vi "GapDetectionNew_nextFour_BM_markus_4.vi"(8 "Sigma in Prozent":dbl=3.0, 9 "Gap":dbl=85.0, 11 "Locations":dbl[](array[numeric])=[1075.5115609583977, 1096.8761989990003, 1148.4828033713086, 1170.9683288122183, 1215.5424277113636]) -> (0 "distanceMatrix":dbl[][](array[numeric])=[[21.364638040602586]], 1 "Array":dbl[](array[numeric]), 2 "FirstGap":dbl=21.364638040602586, 3 "GapPresent":bool)   [LabVIEW 2014]
panel:
  in  "Number of following reflections that should be regarded":i32=1
  in  "probaility higher than":dbl=0.7
  out "exp(x)":dbl[][](array[numeric])
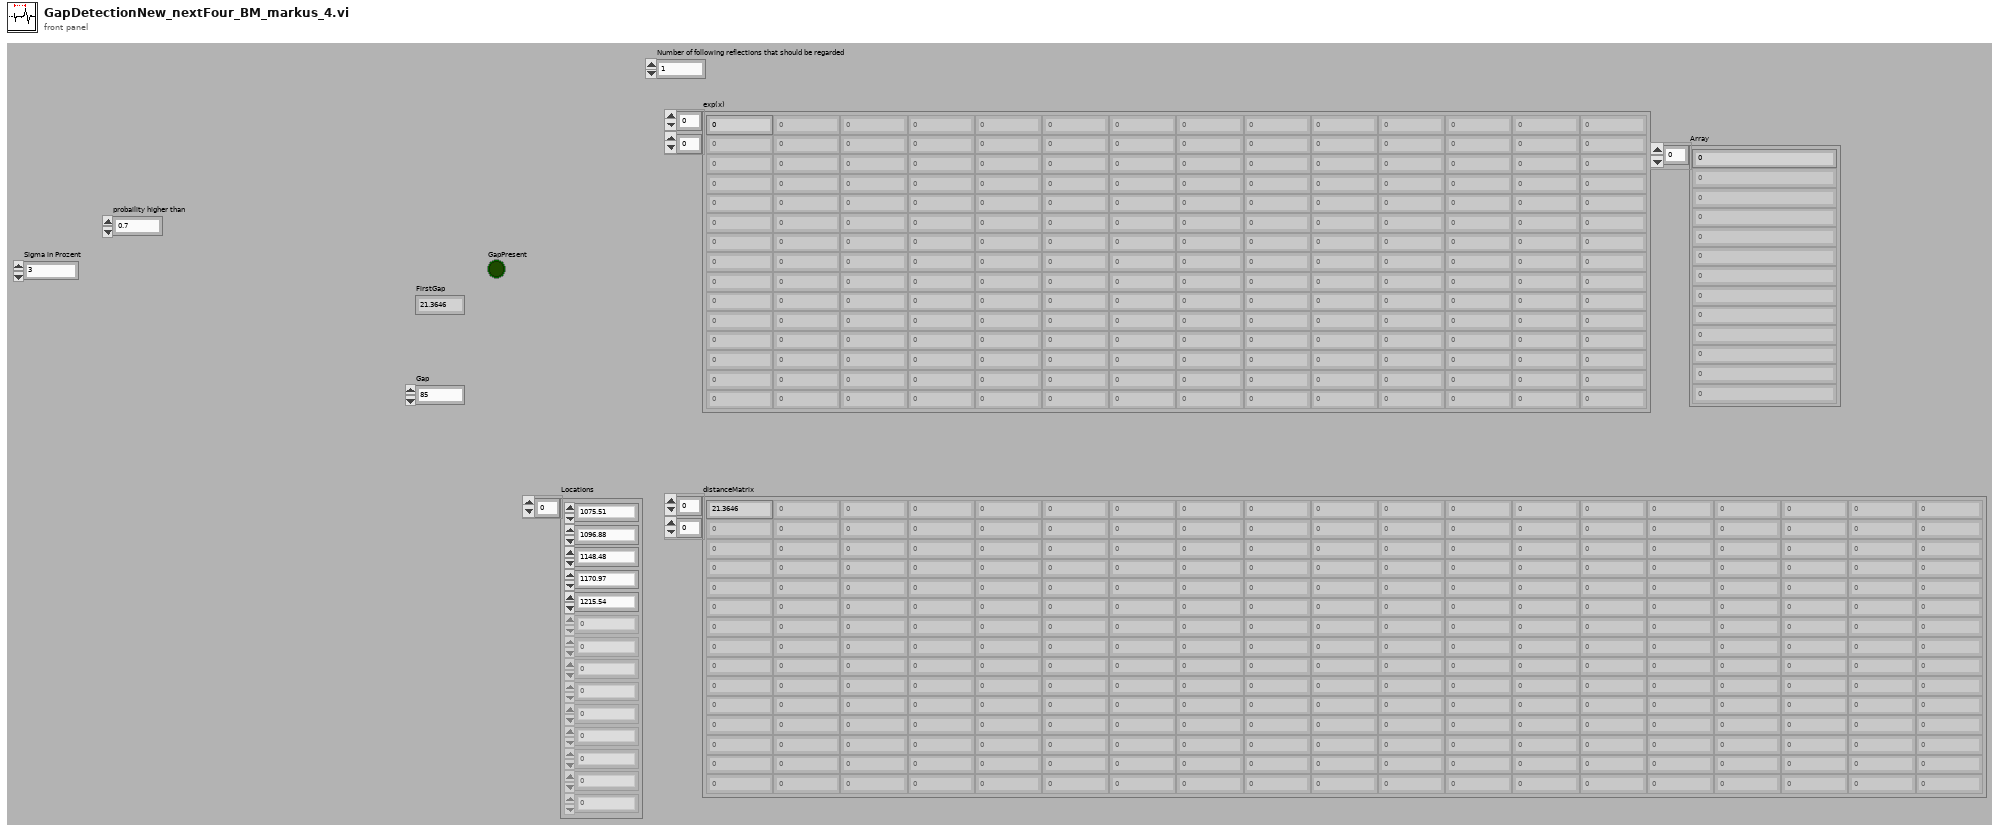
[diagram p1: front panel]
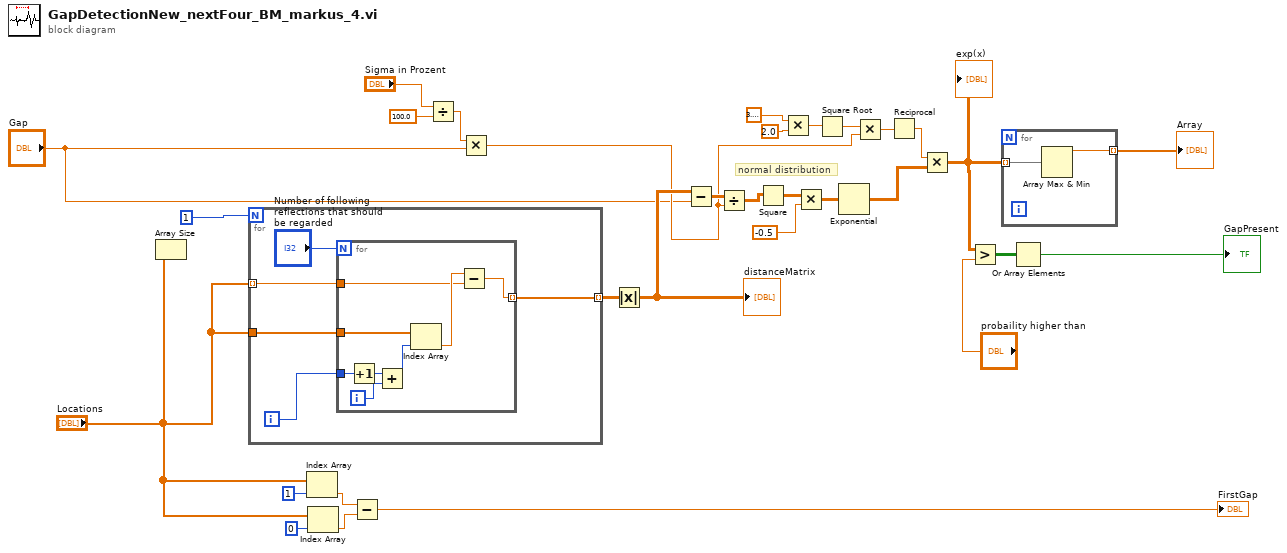
[diagram p0: block diagram]
diagram:
  # "normal distribution"
  n1 = Array Size(array="Locations") -> ()  [unwired: 1 out]
  n2 = for {
    N: 1 -> [_]
    tunnel: [w36] -> w22 mode=indexing
    tunnel: "Locations" -> [w35] mode=indexing
    tunnel: "Locations" -> [w32]
    i -> [w34]
    n3 = for {
      N: "Number of following reflections that should be regarded" -> [_]
      tunnel: [w44] -> w36 mode=indexing
      tunnel: w35 -> [w39]
      tunnel: w34 -> [w38]
      tunnel: w32 -> [w41]
      i -> [w43]
      n4 = Increment(x=w38) -> (x+1=w37:i32)
      n5 = Add(x=w37, y=w43) -> (x+y=w42:i32)
      n6 = Index Array(array=w41, index=w42) -> (element=w40:dbl)
      n7 = Subtract(x=w40, y=w39) -> (x-y=w44:dbl)
    }
  }
  n8 = Index Array(array="Locations", index=1) -> (element=w27:dbl)
  n9 = Index Array(array="Locations", index=0) -> (element=w26:dbl)
  n10 = Subtract(x=w27, y=w26) -> (x-y=→"FirstGap":dbl)
  n11 = Divide(x="Sigma in Prozent", y=100.0) -> (x/y=w9:dbl)
  n12 = Multiply(x=w9, y="Gap") -> (x*y=w7:dbl)
  n13 = Absolute Value(x=w22) -> (abs(x)=w23:dbl[][])
  "distanceMatrix" <- w23
  n14 = Subtract(x=w23, y="Gap") -> (x-y=w17:dbl[][])
  n15 = Divide(x=w17, y=w7) -> (x/y=w16:dbl[][])
  n16 = Square(x=w16) -> (x^2=w15:dbl[][])
  n17 = Multiply(x=3.141592653589793, y=2.0) -> (x*y=w14:dbl)
  n18 = Multiply(x=w15, y=-0.5) -> (x*y=w24:dbl[][])
  n19 = Square Root(x=w14) -> (sqrt(x)=w13:dbl)
  n20 = Exponential(1:w24) -> (0:w3:dbl[][])
  n21 = Multiply(x=w13, y=w7) -> (x*y=w12:dbl)
  n22 = Reciprocal(x=w12) -> (1/x=w4:dbl)
  n23 = Multiply(x=w4, y=w3) -> (x*y=w2:dbl[][])
  "exp(x)" <- w2
  n24 = Greater?(x=w2, y="probaility higher than") -> (0:w20:bool[][])
  n25 = for {
    tunnel: w2 -> [w46] mode=indexing
    tunnel: [w45] -> w10 mode=indexing
    n26 = Array Max & Min(array=w46) -> (max value=w45:dbl)  [unwired: 3 out]
  }
  "Array" <- w10
  n27 = Or Array Elements(Boolean array=w20) -> (logical OR=→"GapPresent":bool)
